vi "ILABs_ViStatus.vi"(2 "errorIn":errorcluster, 3 "name":string, 4 "appReference":refnum<vi>) -> (0 "errorOut":string, 1 "status":i32)   [LabVIEW 2009]
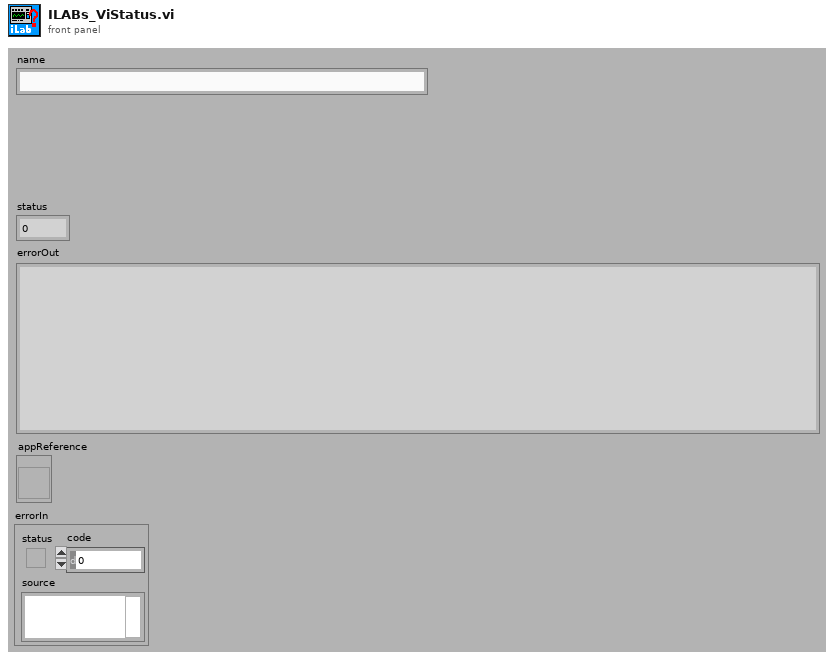
[diagram p1: front panel]
types:
  T1 = enum32{"Bad", "Idle", "Run top level", "Running"}
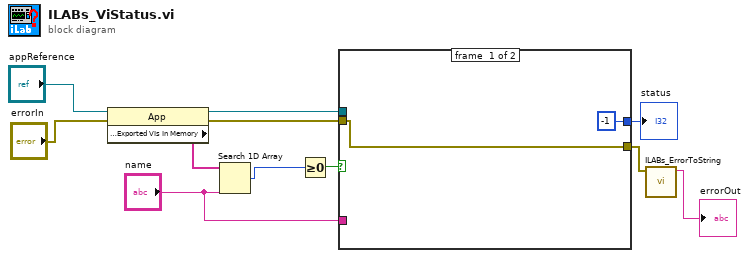
[diagram p0: block diagram]
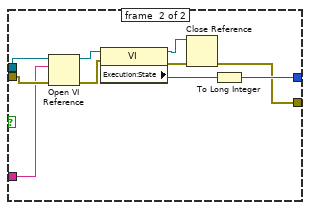
[diagram p2: hidden frame]
diagram:
  n1 = property class="App"(reference="appReference", error in="errorIn") -> (reference out=w7:refnum<vi>, error out=w8:errorcluster, "Application:Exported VIs In Memory"=w11:string[])
  n2 = Search 1D Array(1D array=w11, element="name") -> (index of element=w10:i32)  [unwired: 1 out]
  n3 = Greater Or Equal To 0?(x=w10) -> (x >= 0?=w9:bool)
  n4 = case shown="False" w9 {
    tunnel: w8 -> [w13 w20]
    tunnel: w7 -> [_ w21]
    tunnel: "name" -> [_ w19]
    tunnel: [w13 w14] -> w5
    tunnel: [-1 w17] -> w4
    frame #0 {
    }
    frame #1 {
      n5 = Open VI Reference(application reference (local)=w21, vi path=w19, error in (no error)=w20) -> (vi reference=w23:refnum<vi>, error out=w22:errorcluster)  [unwired: 3 out]
      n6 = property class="VI"(reference=w23, error in=w22) -> (reference out=w16:refnum<vi>, error out=w15:errorcluster, "Execution:State"=w18:T1)
      n7 = Close Reference(reference=w16, error in (no error)=w15) -> (error out=w14:errorcluster)
      n8 = To Long Integer(number=w18) -> (32bit integer=w17:i32)
    }
  }
  "status" <- w4
  n9 = call "ILABs_ErrorToString.vi"("errorIn"=w5) -> ("errorOut"=→"errorOut":string)  [unwired: 10 out]
